vi "Queue.GetReference.vi"(8 "error in (no error)":errorcluster, 11 "queueName":string) -> (0 "error out":errorcluster, 3 "refToQueue":refnum<queue>)   [LabVIEW 2019]
uses:
  QueueMessage.ctl
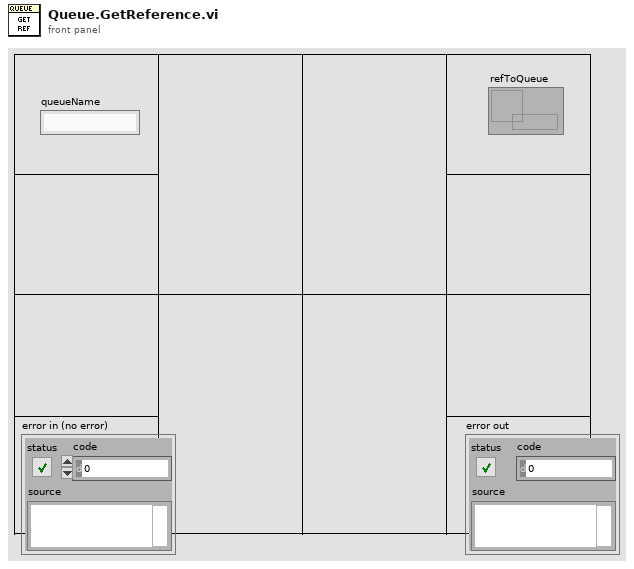
[diagram p1: front panel]
types:
  T1 = typedef "QueueMessage.ctl" = cluster{"message":string, "data":variant}
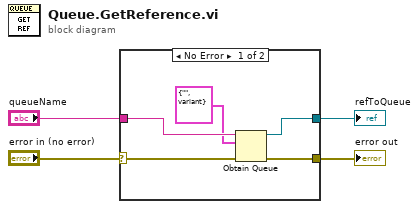
[diagram p0: block diagram]
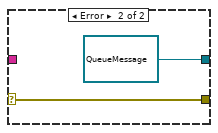
[diagram p2: hidden frame]
diagram:
  n1 = case shown="No Error" "error in (no error)" {
    selector: "error in (no error)" -> [w8 w11]
    tunnel: [w5 w11] -> w1
    tunnel: "queueName" -> [w9 _]
    tunnel: [w6 refnum<queue> refnum ("queue out")] -> w3
    frame No Error {
      n2 = Obtain Queue(name (unnamed)=w9, element data type=T1 {"message"="", "data"=variant} ("QueueMessage"), error in (no error)=w8) -> (queue out=w6:refnum<queue>, error out=w5:errorcluster)  [unwired: 2 in, 1 out]
    }
    frame Error {
    }
  }
  "refToQueue" <- w3
  "error out" <- w1
